vi "Build_Pathname.vi"(1 "Output Array":string[](array[string]), 2 "Pathname":path) -> (0 "Appended path":path)   [LabVIEW 2010]
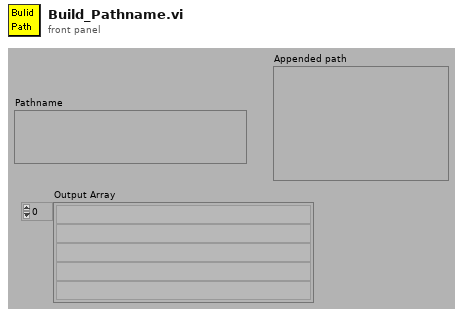
[diagram p1: front panel]
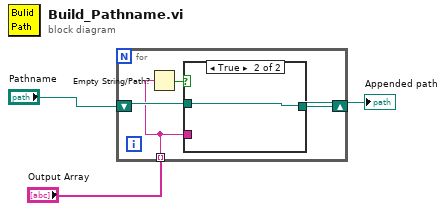
[diagram p0: block diagram]
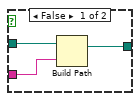
[diagram p2: hidden frame]
diagram:
  n1 = for {
    tunnel: "Output Array" -> [w5] mode=indexing
    shift-right: [w6] -> w1
    shift-left: "Pathname" -> [w7]
    n2 = Empty String/Path?(string/path=w5) -> (empty?=w4:bool)
    n3 = case shown="True" w4 {
      tunnel: w7 -> [w10 w11]
      tunnel: [w9 w11] -> w6
      tunnel: w5 -> [w8 _]
      frame False {
        n4 = Build Path(base path=w10, name or relative path=w8) -> (appended path=w9:path)
      }
      frame True {
      }
    }
  }
  "Appended path" <- w1
